vi "dataUnpackDBLArray.vi"(8 "errorIn":errorcluster, 11 "data":variant) -> (0 "errorOut":errorcluster, 3 "DBLArray":dbl[](array[numeric]))   [LabVIEW 2017]
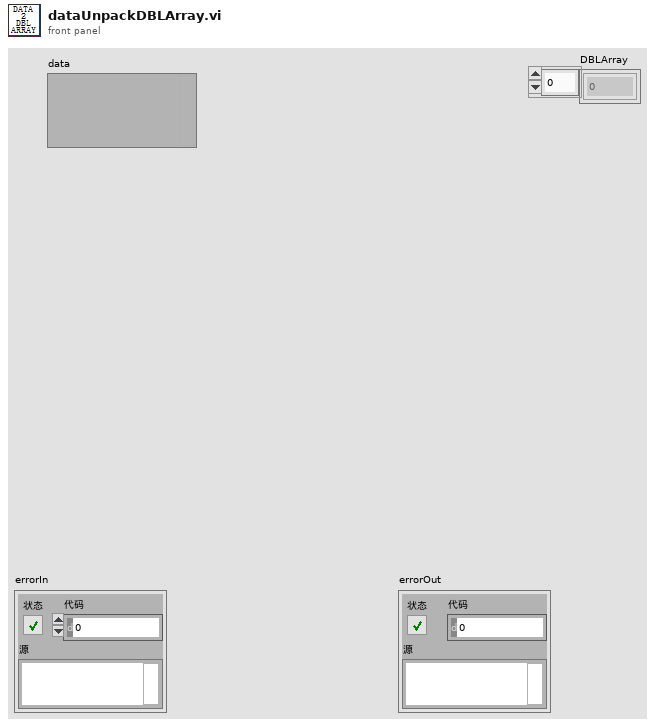
[diagram p1: front panel]
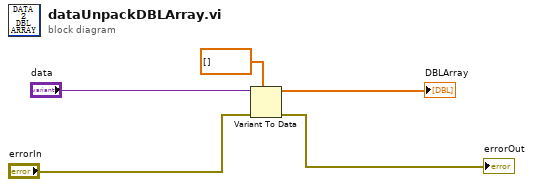
[diagram p0: block diagram]
diagram:
  n1 = Variant To Data(error in="errorIn", type=dbl[] [], Variant="data") -> (data=→"DBLArray":dbl[], error out=→"errorOut":errorcluster)
